vi "SUB-module-StringToArray.vi"(1 "String":string) -> (0 "Arrary":string[](array[string]))   [LabVIEW 2015]
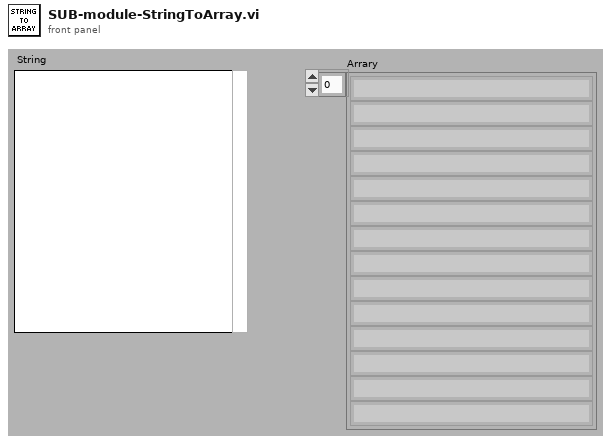
[diagram p1: front panel]
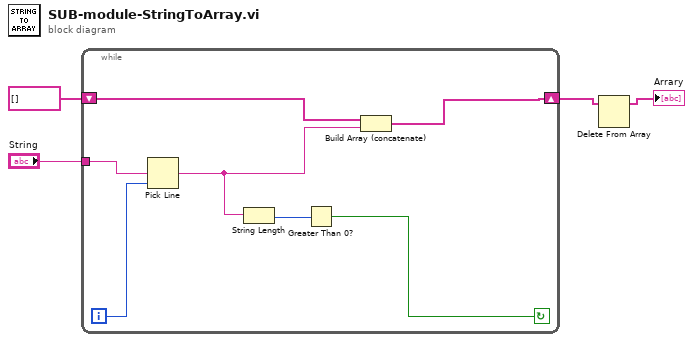
[diagram p0: block diagram]
diagram:
  n1 = while {
    tunnel: "String" -> [w11]
    shift-right: [w9] -> w2
    shift-left: string[] [] -> [w10]
    i -> [w8]
    stop <- w5 continue-if-true
    n2 = Pick Line(multi-line string=w11, line index=w8) -> (output string=w7:string)  [unwired: 1 in]
    n3 = String Length(string=w7) -> (length=w6:i32)
    n4 = Greater Than 0?(x=w6) -> (x > 0?=w5:bool)
    n5 = Build Array (concatenate)(w10, w7) -> (w9:string[])
  }
  n6 = Delete From Array(array=w2) -> (array with subset deleted=→"Arrary":string[])  [unwired: 2 in, 1 out]
